vi "302_Module-DAQ_introduction_Continuous.vi"() -> ()   [LabVIEW 2009]
uses:
  <instrlib>/Zurich Instruments LabOne/Public/Modules/ziTypeModEnum.ctl
  <instrlib>/Zurich Instruments LabOne/Public/Modules/ziModSetValueDoubleArray.vi
  <instrlib>/Zurich Instruments LabOne/Public/Modules/ziModSetValueBinary.vi
  <instrlib>/Zurich Instruments LabOne/Public/Utility/ziTicksToS_vector.vi
  <instrlib>/Zurich Instruments LabOne/Public/Modules/ziModGetDoubleData.vi
  <instrlib>/Zurich Instruments LabOne/Zurich Instruments LabOne.lvlib
panel:
  out "XY Graph":cluster{"Timestamp(s)":dbl[], "Value":dbl[]}[](graph)
  in  "Columns":i32=10 caption="Number of Points"
  in  "Duration":dbl=1.0
  in  "stop":bool
  out "Connected?":bool
  out "Error Out":errorcluster
  in  "Address":string="DEV"
  # "LabOne Modules - DAQ introduction\nThis VI shows how to configure the DAQ module and capture lock-in data. It runs the DAQ module continuously to capture data snapshots with a defined number of points spanned over a defined duration of seconds.\n\nSee block diagram for the VI description.\n\nRequirements: A Zurich Instrument lock-in amplifier\n\nTo run\n1- Type the Instrument ID\n2- Set the sampling duration and number of points.  \n3- Run the VI. It will turn on the signal output of the instrument.\n* You can change Node1 and Value1 Set in the back panel to set different nodes \n\nTested Devices:\n- HF2LI\n- UHFLI\n- MFLI\n\n(c) Zurich Instruments.  ALL RIGHTS RESERVED."
  # "For this VI to work you need to enable the data transfer of the first demodulator in the LabOne user interface"
  # "The Lock-in panel of your instrument might slightly differ depending on the instrument \nand installed options"
  # "The Lock-in panel of your instrument might slightly differ depending on the instrument \nand installed options"
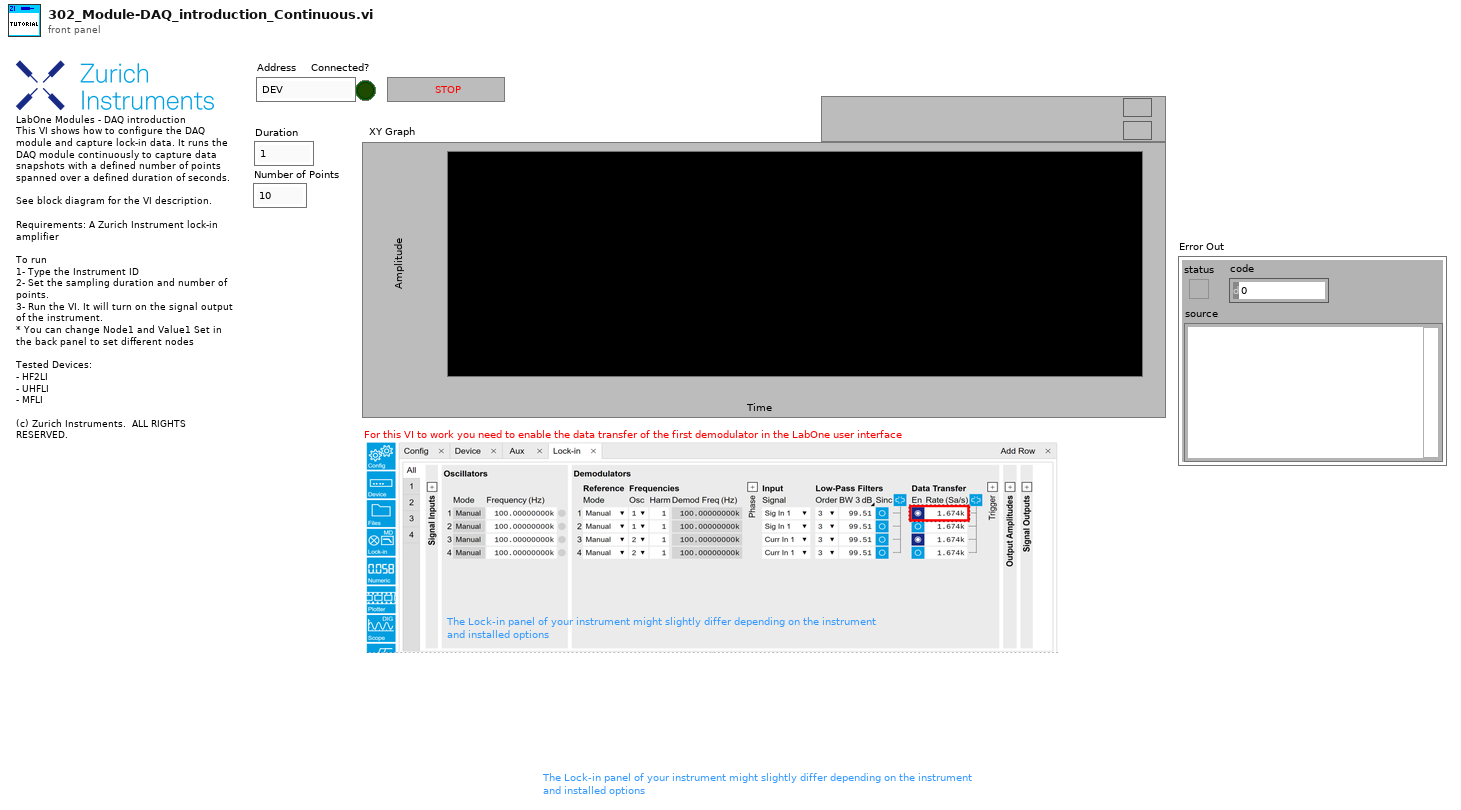
[diagram p1: front panel]
types:
  T1 = typedef "Zurich Instruments LabOne.lvlib/ziTypeModEnum.ctl" = u16
  T2 = typedef "Zurich Instruments LabOne.lvlib/ziTypeHandle.ctl" = cluster{"handleValid":bool, "Conn":u64, "Path Prefix":string, "Handle":u64, "Connected":bool, "Clockbase(s)":dbl}
  T3 = typedef "Zurich Instruments LabOne.lvlib/ziTypeModHandle.ctl" = cluster{"handleValid":bool, "Conn":u64, "ModHandle":u64, "moduleID":string, "Path Prefix":string}
  T4 = cluster{"path":string[], "Value":dbl[][], "Timestamp (ticks)":dbl[][]}
  T5 = typedef "Zurich Instruments LabOne.lvlib/ziTypeModResults.ctl" = cluster{"PathArray":string[], "ValueType":T6, "NoOfResults":u64, "ziGenericHeader":T7[]}
  T6 = typedef "Zurich Instruments LabOne.lvlib/ziTypePollType.ctl" = enum16{"NONE", "DOUBLE_DATA", "INTEGER_DATA", "DEMOD_SAMPLE", "SCOPE_WAVE_HF2", "AUXIN_SAMPLE", "DIO_SAMPLE", "BYTE_ARRAY", "PWA_WAVE", "9", "10", "11", "12", "13", "14", "15", "TREE_CHANGE_DEPRI", "17", "ERROR", "19", "20", "21", "22", "23", "24", "25", "26", "27", "28", "29", "30", "31", "DOUBLE_DATA_TS", "INTEGER_DATA_TS", "34", "SCOPE_WAVE", "SCOPE_WAVE_EX", "37", "BYTE_ARRAY_TS", "39", "40", "41", "42", "43", "44", "45", "CNT_DATA", "47", "TREE_CHANGE", "49", "50", "51", "52", "53", "54", "55", "56", "57", "58", "59", "60", "61", "62", "63", "SWEEPER_DATA", "SPECTRUM_DATA", "ADVISOR_DATA", "VECTOR_DATA", "IMP_DATA", "SHF_GENERATOR_WAVEFORM_DATA", "SHF_RESULT_LOGGER_DATA", "SHF_SCOPE_DATA", "DEMOD_VECTOR"}
  T7 = typedef "Zurich Instruments LabOne.lvlib/ziTypeModGenericHeader.ctl" = cluster{"HeaderType":enum8{"HEADER_TYPE_NONE", "HEADER_TYPE_SWTRIGGER", "HEADER_TYPE_SWEEPER"}, "SampleFormat":u8, "SystemTime":timestamp, "CreatedTimeStamp":u64, "ChangedTimeStamp":u64, "Flags":u32, "ChunkSizeBytes":u64, "Name":string, "Status":u32, "GroupIndex":u32, "Color":u32, "ActiveRow":u32, "TriggerNumber":u64, "GridRows":u32, "GridCols":u32, "GridMode":u32, "GridOperation":u32, "GridDirection":u32, "GridRepetitions":u32, "GridColDelta":dbl, "GridColOffset":dbl, "GridRowDelta":dbl, "GridRowOffset":dbl, "Bandwidth":dbl, "Center":dbl, "Nenbw":dbl}
  T8 = typedef "Zurich Instruments LabOne.lvlib/ziTypeDoubleDataTS.ctl" = cluster{"Timestamp (ticks)":u64[], "Value":dbl[]}
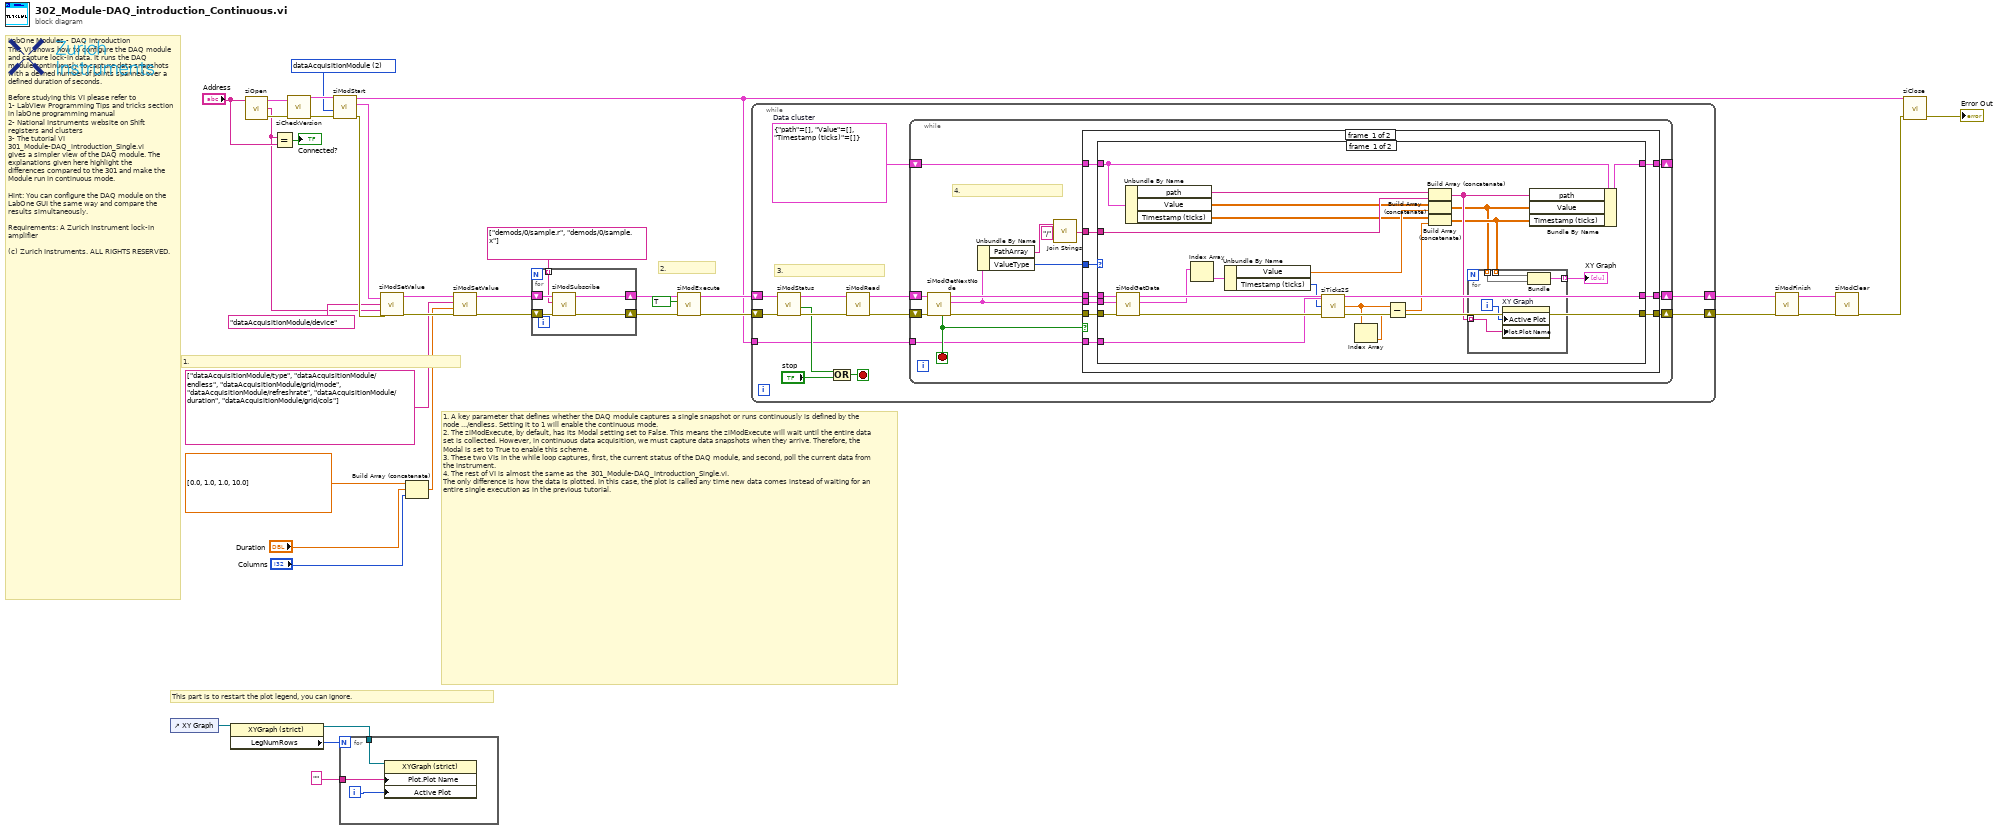
[diagram p0: block diagram]
diagram:
  w30 = T1 2 items=["sweep", "scopeModule", "dataAcquisitionModule", "pidAdvisor", "awgModule", "impedanceModule", "multiDeviceSyncModule", "zoomFFT", "trigger", "deviceSettings", "record"] ("module Id")
  # "2."
  # "This part is to restart the plot legend, you can ignore."
  # "1. A key parameter that defines whether the DAQ module captures a single snapshot or runs continuously is defined by the node .../endless. Setting it to 1 will enable the continuous mode.\n2. The ziModExecute, by default, has its Modal setting set to False. This means the ziModExecute will wait until the entire data set is collected. However, in continuous data acquisition, we must capture data snapshots when they arrive. Therefore, the Modal is set to True to enable this scheme.\n3. These two VIs in the while loop captures, first, the current status of the DAQ module, and second, poll the current data from the instrument.\n4. The rest of VI is almost the same as the  301_Module-DAQ_introduction_Single.vi. \nThe only difference is how the data is plotted. In this case, the plot is called any time new data comes instead of waiting for an entire single execution as in the previous tutorial."
  # "1."
  # "LabOne Modules - DAQ introduction\nThis VI shows how to configure the DAQ module and capture lock-in data. It runs the DAQ module continuously to capture data snapshots with a defined number of points spanned over a defined duration of seconds. \n\nBefore studying this VI please refer to \n1- LabView Programming Tips and tricks section in labOne programming manual\n2- National Instruments website on Shift registers and clusters\n3- The tutorial VI \n301_Module-DAQ_introduction_Single.vi\ngives a simpler view of the DAQ module. The explanations given here highlight the differences compared to the 301 and make the Module run in continuous mode. \n\nHint: You can configure the DAQ module on the LabOne GUI the same way and compare the results simultaneously. \n\nRequirements: A Zurich Instrument lock-in amplifier\n\n(c) Zurich Instruments. ALL RIGHTS RESERVED."
  n1 = control-ref of="XY Graph"() -> (w14:refnum<vi>)
  n2 = property class="XYGraph (strict)"(reference=w14) -> (reference out=w12:refnum<vi>, "LegNumRows"=w13:u32)  [unwired: 1 in, 1 out]
  n3 = call <instrlib>:"ziOpen.vi"("Address"="Address") -> ("Error Out"=w33:errorcluster, "Selected Device"=w26:string, "HandleOut"=w34:T2)  [unwired: 1 in, 2 out]
  n4 = Equal?(x=w26, y="Address") -> (x = y?=→"Connected?":bool)
  n5 = call <instrlib>:"ziCheckVersion.vi"("Handle In"=w34, "Error In"=w33) -> ("Handle Out"=w31:T2, "Error Out"=w32:errorcluster)  [unwired: 11 in, 1 out]
  n6 = call <instrlib>:"ziModStart.vi"("Error In"=w32, "module Id"=w30, "Handle In"=w31) -> ("Error Out"=w28:errorcluster, "ModHandle Out"=w29:T3, "Handle Out"=w1:T2)  [unwired: 6 in]
  n7 = for {
    N: w13 -> [_]
    tunnel: w12 -> [w40]
    tunnel: "" -> [w39]
    i -> [w38]
    n8 = property class="XYGraph (strict)"(reference=w40, "Plot.Plot Name"=w39, "Active Plot"=w38) -> ()  [unwired: 1 in, 2 out]
  }
  n9 = call-poly <instrlib>:"ziModSetValue.vi"("Error In"=w28, "Data"=w26, "Path"="dataAcquisitionModule/device", "ModHandle In"=w29) -> ("Error Out"=w24:errorcluster, "ModHandle Out"=w25:T3)  [unwired: 6 in]
  n10 = Build Array (concatenate)(dbl[] [0.0, 1.0, 1.0, 10.0], "Duration", "Columns") -> (w19:dbl[])
  n11 = call-poly <instrlib>:"ziModSetValue.vi"("Error In"=w24, "Values"=w19, "Paths"=string[] ["dataAcquisitionModule/type", "dataAcquisitionModule/endless", "dataAcquisitionModule/grid/mode", "dataAcquisitionModule/refreshrate", "dataAcquisitionModule/duration", "dataAcquisitionModule/grid/cols"], "ModHandle In"=w25) -> ("Error Out"=w16:errorcluster, "ModHandle Out"=w17:T3)  [unwired: 6 in]
  n12 = for {
    shift-right: [w45] -> w10
    shift-left: w17 -> [w43]
    shift-right: [w44] -> w9
    shift-left: w16 -> [w42]
    tunnel: string[] ["demods/0/sample.r", "demods/0/sample.x"] -> [w41] mode=indexing
    n13 = call <instrlib>:"ziModSubscribe.vi"("Error In"=w42, "Path"=w41, "ModHandle In"=w43) -> ("Error Out"=w44:errorcluster, "ModHandle Out"=w45:T3)  [unwired: 6 in]
  }
  n14 = call <instrlib>:"ziModExecute.vi"("Error In"=w9, "Modal (F)"=TRUE, "ziModHandle In"=w10) -> ("Error Out"=w7:errorcluster, "ziModHandle Out"=w8:T3)  [unwired: 6 in]
  n15 = while {
    tunnel: w1 -> [w46]
    shift-right: [w48] -> w5
    shift-left: w8 -> [w55]
    shift-right: [w47] -> w4
    shift-left: w7 -> [w54]
    stop <- w56 stop-if-true
    w58 = T4 {"path"=[], "Value"=[], "Timestamp (ticks)"=[]}  # Data cluster
    # "3."
    n16 = call <instrlib>:"ziModStatus.vi"("Error In"=w54, "ModHandle IN"=w55) -> ("Error Out"=w52:errorcluster, "Finished?"=w49:bool, "ModHandle Out"=w53:T3)  [unwired: 5 in, 1 out]
    n17 = Compound Arithmetic op=OR(w49, "stop") -> (w56:bool)
    n18 = call <instrlib>:"ziModRead.vi"("error in"=w52, "ziModHandle In"=w53) -> ("error out"=w50:errorcluster, "ziModHandle Out"=w51:T3)  [unwired: 8 in]
    n19 = while {
      shift-right: [w65] -> _
      shift-left: w58 -> [w66]
      tunnel: w46 -> [w59]
      shift-right: [w60] -> w48
      shift-left: w51 -> [w72]
      shift-right: [w61] -> w47
      shift-left: w50 -> [w73]
      stop <- w71 stop-if-true
      # "4."
      n20 = call <instrlib>:"ziModGetNextNode.vi"("Error In"=w73, "ModHandle In"=w72) -> ("Error Out"=w70:errorcluster, "ModResults"=w68:T5, "ModHandle Out"=w69:T3, "NoData"=w71:bool)  [unwired: 6 in]
      n21 = Unbundle By Name(w68) -> ("PathArray"=w63:string[], "ValueType"=w67:T6)
      n22 = call <vilib>:"Join Strings.vi"("Separator (,)"="/", "Strings In"=w63) -> ("String"=w62:string)  [unwired: 1 in]
      n23 = case shown="False" w71 {
        tunnel: w70 -> [w81 w117]
        tunnel: w69 -> [w82 w118]
        tunnel: [w79 w118] -> w60
        tunnel: [w80 w117] -> w61
        tunnel: w68 -> [w83 _]
        tunnel: w67 -> [w78 _]
        tunnel: [w77 w116] -> w65
        tunnel: w66 -> [w76 w116]
        tunnel: w62 -> [w75 _]
        tunnel: w59 -> [w74 _]
        frame #0 {
          n24 = case shown="\"DOUBLE_DATA_TS\"" w78 {
            tunnel: w83 -> [w107 _]
            tunnel: w82 -> [w106 w114]
            tunnel: w81 -> [w105 w113]
            tunnel: [w96 w113] -> w80
            tunnel: [w104 w114] -> w79
            tunnel: [w100 w115] -> w77
            tunnel: w76 -> [w101 w115]
            tunnel: w75 -> [w98 _]
            tunnel: w74 -> [w95 _]
            frame #0 {
              n25 = call-poly <instrlib>:"ziModGetData.vi"("Error In"=w105, "ModResults"=w107, "ModHandle In"=w106) -> ("Error Out"=w97:errorcluster, "DoubleSample"=w103:T8[], "ModHandle Out"=w104:T3)  [unwired: 4 in, 2 out]
              n26 = Unbundle By Name(w101) -> ("path"=w99:string[], "Value"=w87:dbl[][], "Timestamp (ticks)"=w85:dbl[][])
              n27 = Index Array(array=w103) -> (element=w102:T8)  [unwired: 1 in]
              n28 = Unbundle By Name(w102) -> ("Value"=w91:dbl[], "Timestamp (ticks)"=w94:u64[])
              n29 = call-poly <instrlib>:"ziTicks2S.vi"("Error In"=w97, "Timestamp (ticks)"=w94, "Handle In"=w95) -> ("Error Out"=w96:errorcluster, "Timestamp(s)"=w92:dbl[])  [unwired: 1 out]
              n30 = Index Array(array=w92) -> (element=w93:dbl)  [unwired: 1 in]
              n31 = Subtract(x=w92, y=w93) -> (x-y=w90:dbl[])
              n32 = Build Array (concatenate)(w99, w98) -> (w89:string[])
              n33 = Build Array (concatenate)(w87, w91) -> (w84:dbl[][])
              n34 = Build Array (concatenate)(w85, w90) -> (w86:dbl[][])
              n35 = for {
                tunnel: [w112] -> w88 mode=indexing
                tunnel: w89 -> [w108] mode=indexing
                tunnel: w86 -> [w111] mode=indexing
                tunnel: w84 -> [w110] mode=indexing
                i -> [w109]
                n36 = property on="XY Graph" class="XYGraph (strict)"("Active Plot"=w109, "Plot.Plot Name"=w108) -> ()  [unwired: 2 in, 2 out]
                n37 = Bundle(w111, w110) -> (w112:cluster{dbl[], dbl[]})  [unwired: 1 in]
              }
              "XY Graph" <- w88
              n38 = Bundle By Name(cluster=w101, "path"=w89, "Value"=w84, "Timestamp (ticks)"=w86) -> (w100:T4)
            }
            frame #1 {
            }
          }
        }
        frame #1 {
        }
      }
    }
  }
  n39 = call <instrlib>:"ziModFinish.vi"("Error In"=w4, "ziModHandle In"=w5) -> ("Error Out"=w2:errorcluster, "ziModHandle Out"=w3:T3)  [unwired: 7 in]
  n40 = call <instrlib>:"ziModClear.vi"("Error In"=w2, "ziModHandle In"=w3) -> ("Error Out"=w18:errorcluster)  [unwired: 7 in, 1 out]
  n41 = call <instrlib>:"ziClose.vi"("Error In"=w18, "Handle In"=w1) -> ("Error Out"=→"Error Out":errorcluster)  [unwired: 2 in, 1 out]
